vi "Write VacuumLines Obj.vi"(8 "error in (no error)":errorcluster, 10 "Hardware.lvlib:VacuumLine.lvlib:VacuumLines.lvclass":refnum<class "VacuumLines.lvclass">, 11 "VacuumLines Configuration in":refnum<class "VacuumLines Configuration.lvclass">) -> (0 "error out":errorcluster, 3 "VacuumLines Configuration out":refnum<class "VacuumLines Configuration.lvclass">)   [LabVIEW 2016, in "Hardware.lvlib" / "VacuumLine.lvlib" / "VacuumLines Configuration.lvclass"]
uses:
  <userlib>/Common Components/Hardware/Abstract System/VacuumLine/VacuumLines Configuration/VacuumLines Configuration.lvclass
  <userlib>/Common Components/Hardware/Abstract System/VacuumLine/VacuumLines/VacuumLines.lvclass
  <userlib>/Common Components/Hardware/Abstract System/VacuumLine/VacuumLines Configuration/VacuumLines Configuration.lvclass/VacuumLines Configuration.ctl
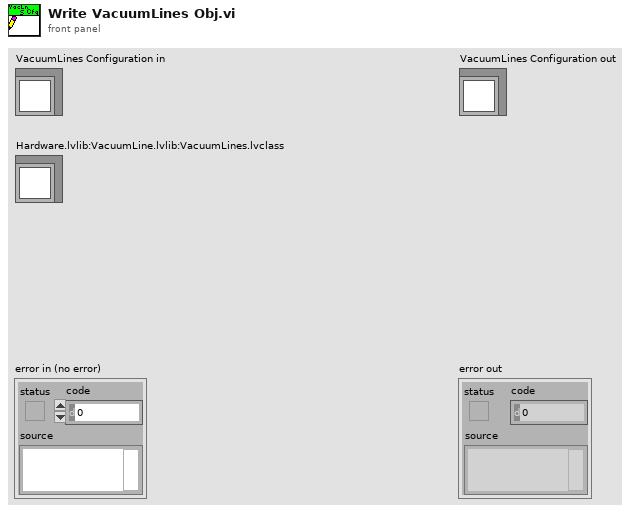
[diagram p1: front panel]
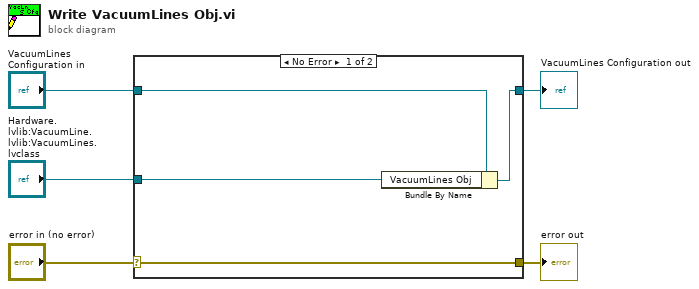
[diagram p0: block diagram]
diagram:
  n1 = case shown="No Error" "error in (no error)" {
    selector: "error in (no error)" -> [w9 w10]
    tunnel: [w9 w10] -> w4
    tunnel: [w7 w11] -> w2
    tunnel: "VacuumLines Configuration in" -> [w8 w11]
    tunnel: "Hardware.lvlib:VacuumLine.lvlib:VacuumLines.lvclass" -> [w6 _]
    frame No Error {
      n2 = Bundle By Name(cluster=w8, "VacuumLines Obj"=w6) -> (w7:refnum<class "VacuumLines Configuration.lvclass">)
    }
    frame Error {
    }
  }
  "error out" <- w4
  "VacuumLines Configuration out" <- w2
